vi "VoltageTest_L_VDC5V.vi"(0 "datain":string[](array[string])=["备注", "负载通道", "负载地址", "延时时间", "output max", "output min", "量测类型", "待测物板号"], 5 "HW CH Number":i32, 7 "Setup":string) -> (4 "REPORT INDECATE":string[][](array[string])=[["微安测试", "", "", "", ""], ["微安量测", "4", "0.000", "0.1", "NG"], ["微安量测", "4", "0.000", "0.1", "NG"], ["微安量测", "4", "0.000", "0.1", "NG"], ["微安量测", "4", "0.000", "0.1", "NG"]], 6 "ROW HEAD":string[](array[string]), 8 "PF":string[](array[string]), 10 "testData":string[](array[string]), 15 "Array":string[](array[string]))   [LabVIEW 2018]
uses:
  Subvi/Global.vi
panel:
  out "测试板数":i32
  out "数组":bool[](array[boolean])
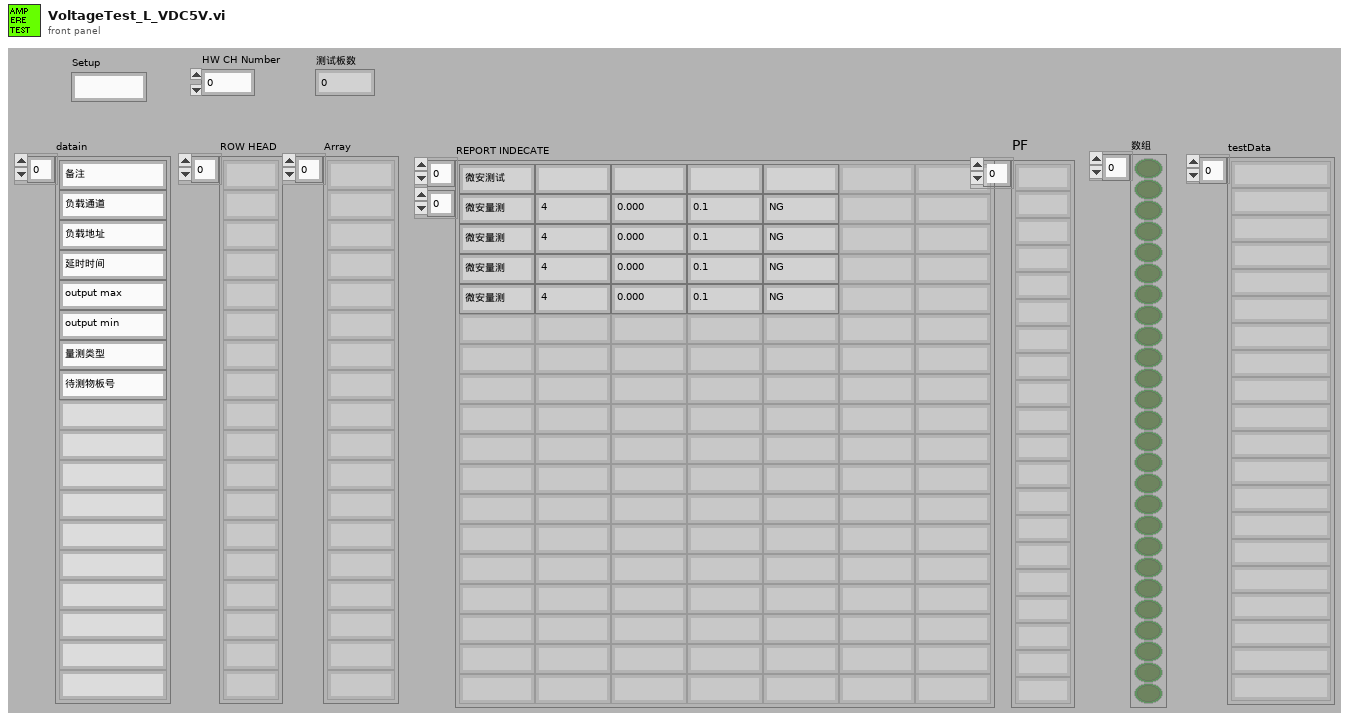
[diagram p1: front panel]
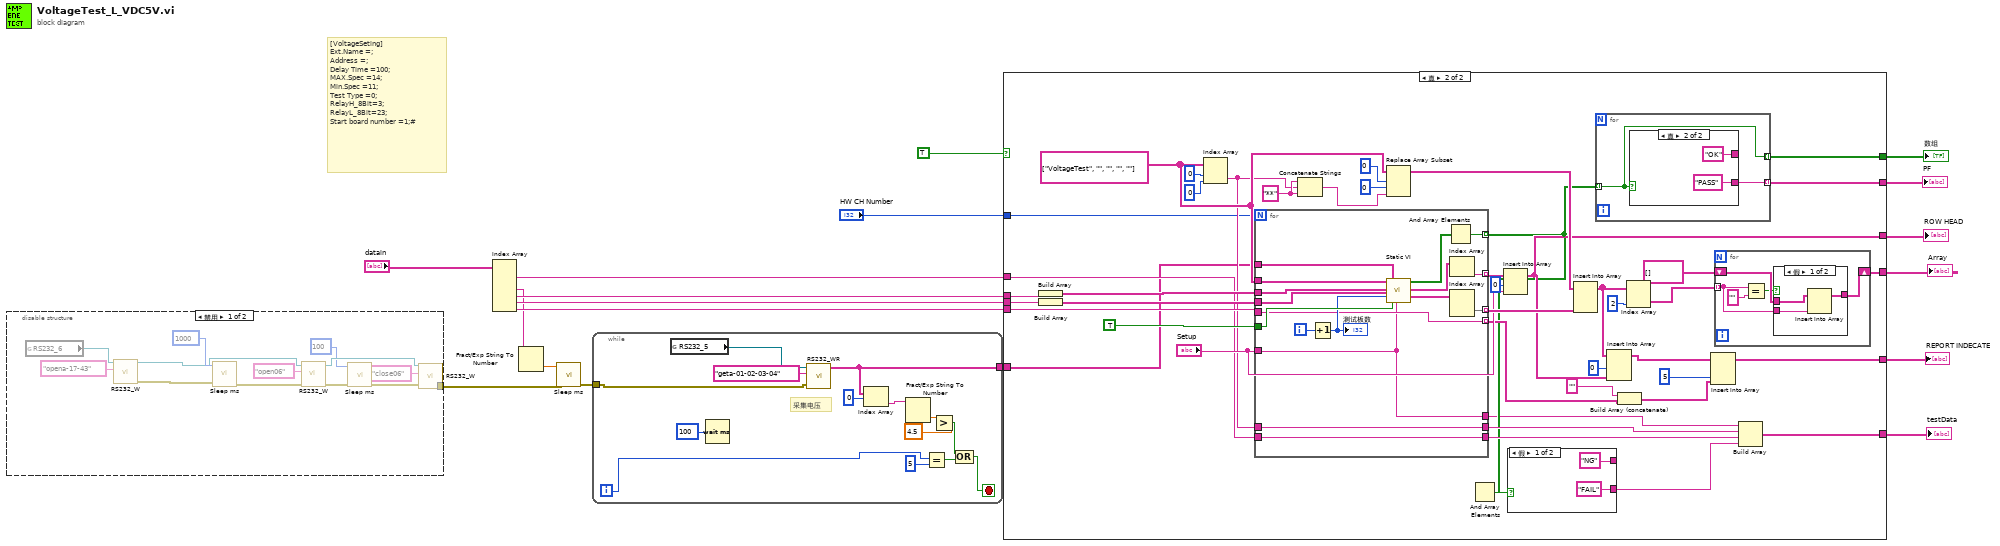
[diagram p0: block diagram]
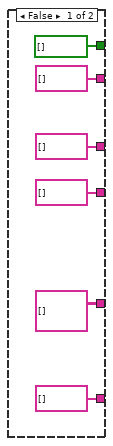
[diagram p3: hidden frame]
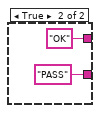
[diagram p4: hidden frame]
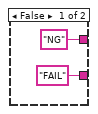
[diagram p5: hidden frame]
diagram:
  # "[VoltageSeting]\nExt.Name =;\nAddress =;\nDelay Time =100;\nMAX.Spec =14;\nMin.Spec =11;\nTest Type =0;\nRelayH_8Bit=3;\nRelayL_8Bit=23;\nStart board number =1;#"
  n1 = disable-structure shown="禁用" {
    disable-tunnel: [w23 _] -> w3
    frame Disabled {
      n2 = global read "Global.vi" "RS232_6"() -> (w22:refnum<visa-resource-name>)
      n3 = call "RS232_W.vi"("CMD"="opena-17-43", "VISA资源名称"=w22) -> ("error out"=w19:errorcluster, "VISA资源名称输出"=w20:refnum<visa-resource-name>)  [unwired: 7 in, 1 out]
      n4 = call "Sleep ms.vi"("error in (no error)"=w19, "等待时间（毫秒）"=u32 1000) -> ("error out"=w30:errorcluster)  [unwired: 9 in]
      n5 = call "RS232_W.vi"("error in (no error)"=w30, "CMD"="open06", "VISA资源名称"=w20) -> ("error out"=w25:errorcluster, "VISA资源名称输出"=w29:refnum<visa-resource-name>)  [unwired: 6 in, 1 out]
      n6 = call "Sleep ms.vi"("error in (no error)"=w25, "等待时间（毫秒）"=u32 100) -> ("error out"=w28:errorcluster)  [unwired: 9 in]
      n7 = call "RS232_W.vi"("error in (no error)"=w28, "CMD"="close06", "VISA资源名称"=w29) -> ("error out"=w23:errorcluster)  [unwired: 6 in, 2 out]
    }
    frame Enabled {
    }
  }
  n8 = Index Array(array="datain") -> (element #1=w10:string, element #3=w2:string, element #4=w15:string, element #5=w14:string, element #6=w12:string)  [unwired: 6 in, 1 out]
  n9 = Fract/Exp String To Number(string=w2) -> (number=w4:dbl)  [unwired: 3 in, 1 out]
  n10 = call "Sleep ms.vi"("error in (no error)"=w3, "等待时间（毫秒）"=w4) -> ("error out"=w1:errorcluster)  [unwired: 9 in]
  n11 = while {
    tunnel: [w36] -> w6
    tunnel: w1 -> [w33]
    i -> [w35]
    stop <- w34 stop-if-true
    # "采集电压"
    n12 = global read "Global.vi" "RS232_5"() -> (w44:refnum<visa-resource-name>)
    n13 = Wait (ms)(milliseconds to wait=u32 100 ("等待时间（毫秒）")) -> ()  [unwired: 1 out]
    n14 = call "RS232_WR.vi"("error in (no error)"=w33, "CMD"="geta-01-02-03-04", "VISA资源名称"=w44) -> ("Out data"=w36:string[])  [unwired: 6 in, 2 out]
    n15 = Index Array(array=w36, index=0 ("索引")) -> (element=w42:string)
    n16 = Fract/Exp String To Number(string=w42) -> (number=w41:dbl)  [unwired: 3 in, 1 out]
    n17 = Equal?(x=w35, y=5) -> (x = y?=w43:bool)
    n18 = Greater?(x=w41, y=4.5) -> (0:w40:bool)
    n19 = Compound Arithmetic op=OR ("复合运算")(w40, w43) -> (w34:bool)
  }
  n20 = case shown="真" TRUE {
    tunnel: [string[] [] ("Array") w92] -> w18
    tunnel: [string[] [] w91] -> w17
    tunnel: w15 -> [_ w84]
    tunnel: w14 -> [_ w83]
    tunnel: [string[] [] w72] -> w13
    tunnel: w12 -> [_ w70]
    tunnel: [string[][] [] w67] -> w11
    tunnel: w10 -> [_ w62]
    tunnel: [string[] [] w56] -> w9
    tunnel: [bool[] [] w54] -> w8
    tunnel: "HW CH Number" -> [_ w53]
    tunnel: w6 -> [_ w52]
    frame False {
    }
    frame True {
      w82 = string[][] [["VoltageTest", "", "", "", ""]]
      w88 = "**" ("字符串")
      n21 = Build Array(w84) -> (w81:string[])
      n22 = Build Array(w83) -> (w80:string[])
      n23 = Index Array(array=w82, index (row)=0 ("索引 (行)"), index (col)=0 ("禁用的索引 (列)")) -> (element=w63:string)
      n24 = for {
        N: w53 -> [_]
        tunnel: w52 -> [w116]
        tunnel: w81 -> [w114]
        tunnel: w80 -> [w113]
        tunnel: "Setup" -> [w100]
        tunnel: TRUE -> [w111]
        tunnel: [w109] -> w58 mode=indexing
        tunnel: [w106] -> w76 mode=indexing
        tunnel: w82 -> [w115]
        tunnel: [w104] -> w77 mode=indexing
        tunnel: w70 -> [w103]
        tunnel: [w103] -> w66 mode=indexing
        tunnel: w63 -> [w102]
        tunnel: [w102] -> w61
        tunnel: w62 -> [w101]
        tunnel: [w101] -> w60
        tunnel: [w100] -> w55
        i -> [w108]
        n25 = Increment(x=w108) -> (x+1=w110:i32)
        "测试板数" <- w110
        n26 = call "Static VI.vi"("添加的数组"=w115, "Max"=w114, "Min"=w113, "板数"=w110, "INPUTSTRING"=w116, "是否为字符串对比"=w111, "SQ"=w100) -> ("P/F"=w112:bool[], "SQ out"=w107:string[], "arrauy out"=w105:string[][])  [unwired: 9 in, 1 out]
        n27 = And Array Elements(Boolean array=w112) -> (logical AND=w109:bool)
        n28 = Index Array(array=w107) -> (element=w106:string)  [unwired: 1 in]
        n29 = Index Array(array=w105) -> (element=w104:string[])  [unwired: 2 in]
      }
      n30 = Concatenate Strings(w88, w63, w88) -> (w85:string)
      n31 = Replace Array Subset(array=w82, new element=w85, index (row)=0 ("索引 (行)"), index (col)=0 ("禁用的索引 (列)")) -> (w78:string[][])
      n32 = And Array Elements(Boolean array=w58) -> (logical AND=w59:bool)
      n33 = Insert Into Array(array=w76, index=0 ("索引"), new element="Setup") -> (w72:string[])
      n34 = case shown="假" w59 {
        tunnel: ["NG" "OK"] -> _
        tunnel: ["FAIL" "PASS"] -> w57
        frame False {
        }
        frame True {
        }
      }
      n35 = Insert Into Array ("数组插入")(array=w78, new element=w77) -> (w73:string[][])  [unwired: 2 in]
      n36 = for {
        tunnel: w58 -> [w117] mode=indexing
        tunnel: [w118] -> w91 mode=indexing
        tunnel: [w117] -> w54 mode=indexing
        n37 = case shown="真" w117 {
          tunnel: ["NG" "OK"] -> _
          tunnel: ["FAIL" "PASS"] -> w118
          frame False {
          }
          frame True {
          }
        }
      }
      n38 = Insert Into Array(array=w73, index (col)=0 ("禁用的索引 (列)"), new element=w72) -> (w68:string[][])  [unwired: 1 in]
      n39 = Build Array (concatenate)("" ("字符串"), w66) -> (w64:string[])
      n40 = Index Array(array=w73, index (col)=2 ("禁用的索引 (列)")) -> (element=w93:string[])  [unwired: 1 in]
      n41 = Insert Into Array(array=w68, index (col)=5 ("禁用的索引 (列)"), new element=w64) -> (w67:string[][])  [unwired: 1 in]
      n42 = for {
        tunnel: w93 -> [w123] mode=indexing
        shift-right: [w124] -> w92
        shift-left: string[] [] ("Array") -> [w127]
        n43 = Equal?(x=w123, y="") -> (x = y?=w125:bool)
        n44 = case shown="假" w125 {
          tunnel: w127 -> [w130 w131]
          tunnel: [w129 w131] -> w124
          tunnel: w123 -> [w128 _]
          frame False {
            n45 = Insert Into Array(array=w130, new element=w128) -> (w129:string[])  [unwired: 1 in]
          }
          frame True {
          }
        }
      }
      n46 = Build Array(w55, w61, w60, w57) -> (w56:string[])
    }
  }
  "REPORT INDECATE" <- w11
  "ROW HEAD" <- w13
  "PF" <- w17
  "Array" <- w18
  "数组" <- w8
  "testData" <- w9
